vi "DAQ Loop.vi"(8 "error in":errorcluster, 10 "Queues":T1, 11 "Notifiers":T2) -> (0 "error out":errorcluster)   [LabVIEW 2014, in "DAQ.lvlib"]
uses:
  DAQ.lvlib
  support/Message Queue/Message Queue.lvlib
  TypeDefs/DAQ data.ctl
  <vilib>/ErrorRing/Error Ring.xnode
  PLC/PLC.lvlib
  support/Global names.vi
  <vilib>/Utility/error.llb/Error Cluster From Error Code.vi
  support/Message Queue/Message Cluster.ctl
  support/Notifiers/Notifiers.ctl
  Support/Notifiers/Notifiers.lvlib
  support/Message Queue/All Message Queues.ctl
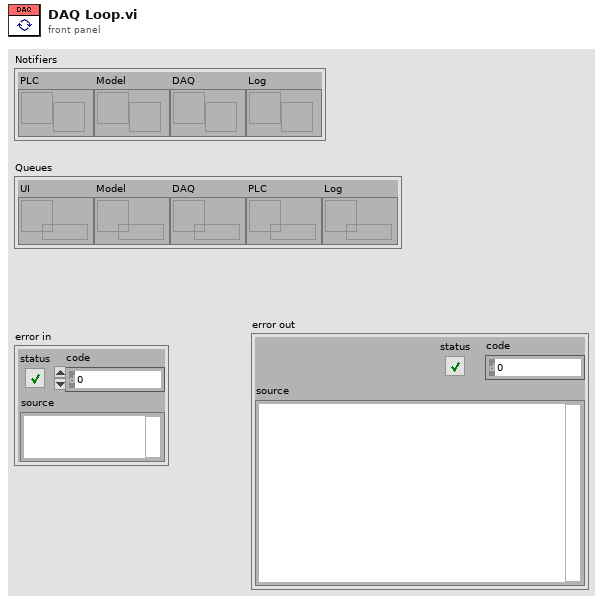
[diagram p1: front panel]
types:
  T1 = typedef "Message Queue.lvlib/All Message Queues.ctl" = cluster{"UI":refnum<queue>, "Model":refnum<queue>, "DAQ":refnum<queue>, "PLC":refnum<queue>, "Log":refnum<queue>}
  T2 = typedef "Notifiers.lvlib/Notifiers.ctl" = cluster{"PLC":refnum<notifier>, "Model":refnum<notifier>, "DAQ":refnum<notifier>, "Log":refnum<notifier>}
  T3 = typedef "DAQ.lvlib/DAQ data.ctl" = cluster{"Power switch (DI)":cluster{"Channel":tag, "Data":bool}, "Dispose barrel (DI)":cluster{"Channel":tag, "Data":bool}, "Pump status (DO)":cluster{"Channel":tag, "Data":bool}, "Barrel position (AI)":cluster{"Channel":tag, "Data":dbl}}
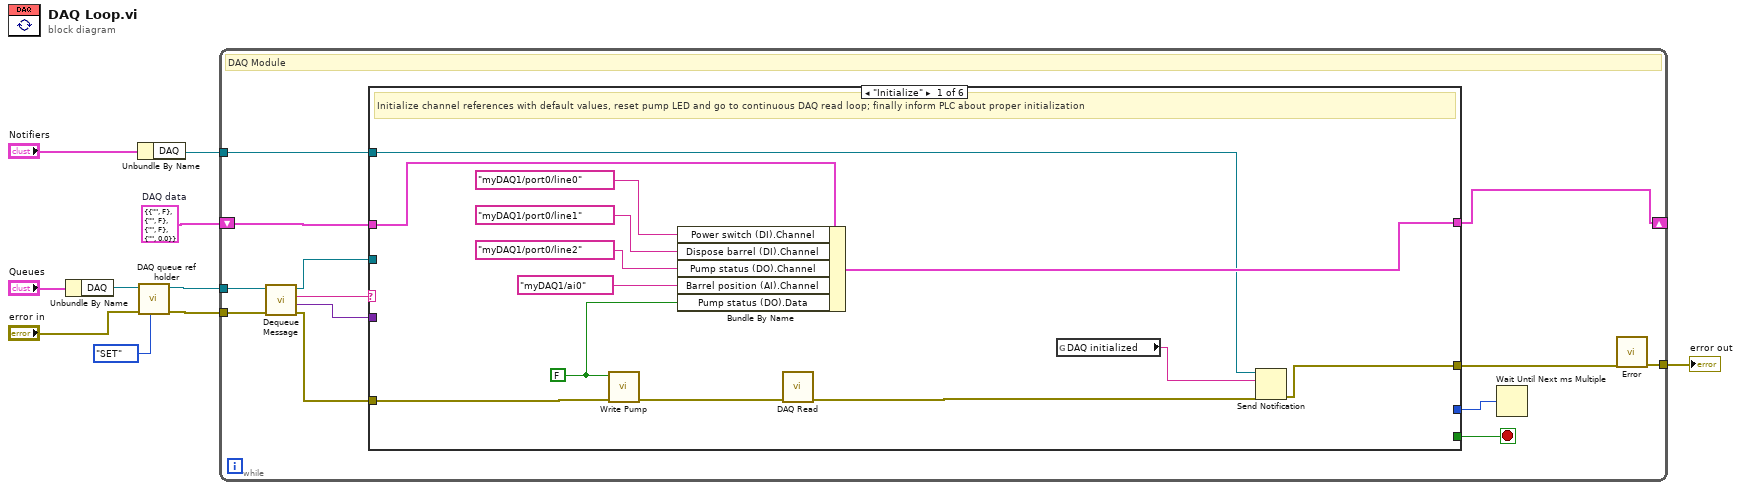
[diagram p0: block diagram]
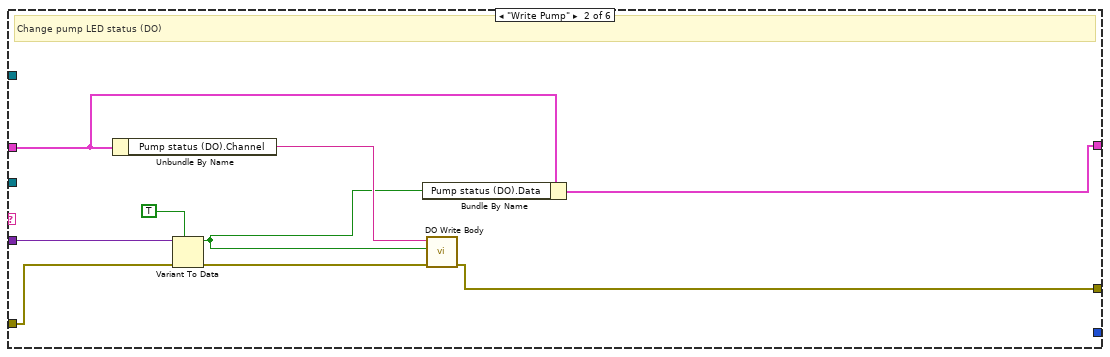
[diagram p2: hidden frame]
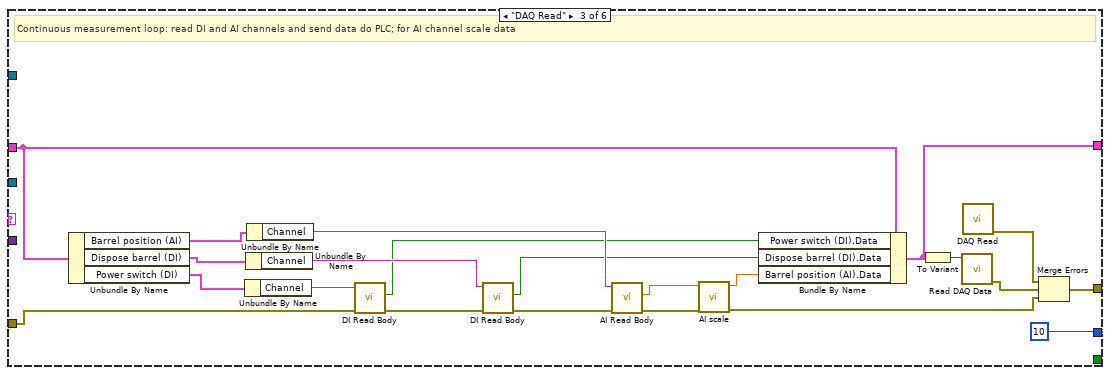
[diagram p3: hidden frame]
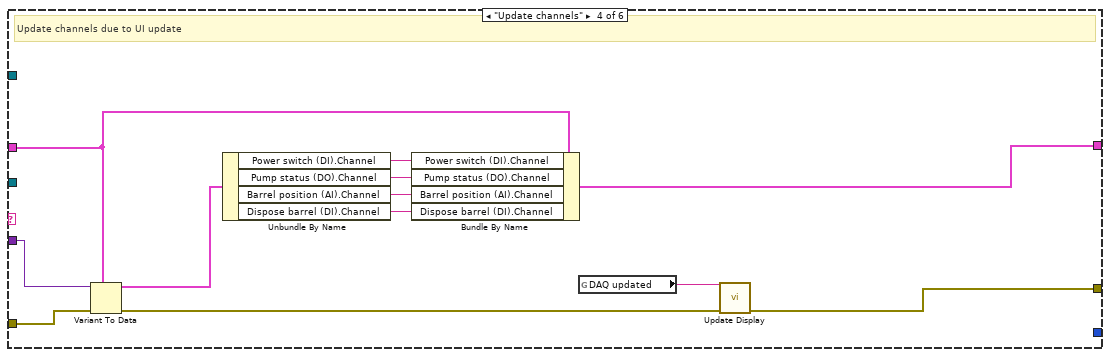
[diagram p4: hidden frame]
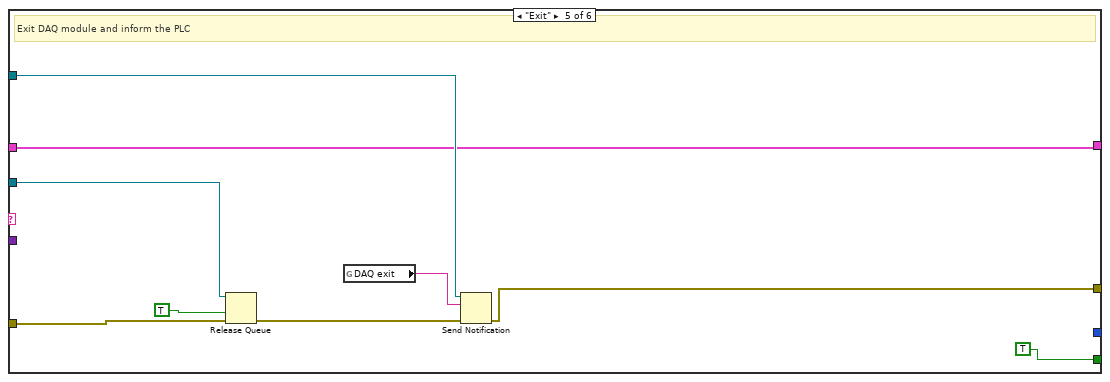
[diagram p5: hidden frame]
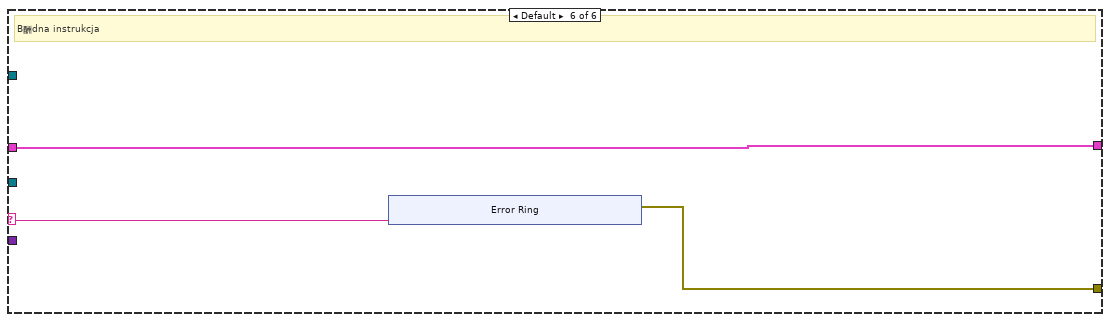
[diagram p6: hidden frame]
diagram:
  w10 = T3 {"Power switch (DI)"={"Channel"="", "Data"=FALSE}, "Dispose barrel (DI)"={"Channel"="", "Data"=FALSE}, "Pump status (DO)"={"Channel"="", "Data"=FALSE}, "Barrel position (AI)"={"Channel"="", "Data"=0.0}}  # DAQ data
  n1 = Unbundle By Name("Queues") -> ("DAQ"=w5:refnum<queue>)
  n2 = Unbundle By Name("Notifiers") -> ("DAQ"=w6:refnum<notifier>)
  n3 = call "DAQ queue ref holder.vi"("Action"=enum16{"GET", "SET"}."SET", "error in"="error in", "Message Queue In"=w5) -> ("error out"=w3:errorcluster, "Input Message Queue"=w4:refnum<queue>)  [unwired: 7 in]
  n4 = while {
    tunnel: w3 -> [w23]
    tunnel: w4 -> [w11]
    tunnel: w6 -> [w19]
    shift-right: [w18] -> _
    shift-left: w10 -> [w16]
    tunnel: [w14] -> w8
    stop <- w20 stop-if-true
    # "DAQ Module"
    n5 = call "Dequeue Message.vi"("error in (no error)"=w23, "Message Queue"=w11) -> ("error out"=w22:errorcluster, "Message Data"=w21:variant, "Message"=w12:string, "dup Message Queue"=w13:refnum<queue>)  [unwired: 6 in]
    n6 = case shown="\"Initialize\"" w12 {
      selector: w12 -> [_ _ _ _ _ w90]
      tunnel: w22 -> [w29 w45 w54 w78 w82 _]
      tunnel: [w35 w37 w49 w70 w81 w89] -> w15
      tunnel: w21 -> [_ w44 _ w79 _ _]
      tunnel: [_ _ _ _ TRUE _] -> w20
      tunnel: w13 -> [_ _ _ _ w88 _]
      tunnel: w19 -> [w27 _ _ _ w87 _]
      tunnel: w16 -> [w34 w41 w64 w77 w83 w91]
      tunnel: [w33 w43 w58 w72 w83 w91] -> w18
      tunnel: [_ _ u32 10 ("millisecond multiple") _ _ _] -> w17
      frame "Initialize" {
        w26 = FALSE
        # "Initialize channel references with default values, reset pump LED and go to continuous DAQ read loop; finally inform PLC about proper initialization"
        n7 = call "Write Pump.vi"("error in"=w29, "Pump state"=w26) -> ("error out"=w28:errorcluster)  [unwired: 9 in]
        n8 = Bundle By Name(cluster=w34, "Power switch (DI).Channel"=tag "myDAQ1/port0/line0", "Dispose barrel (DI).Channel"=tag "myDAQ1/port0/line1" ("Power switch (DI).Channel"), "Pump status (DO).Channel"=tag "myDAQ1/port0/line2" ("Power switch (DI).Channel"), "Barrel position (AI).Channel"=tag "myDAQ1/ai0", "Pump status (DO).Data"=w26) -> (w33:T3)
        n9 = call "DAQ Read.vi"("error in"=w28) -> ("error out"=w25:errorcluster)  [unwired: 10 in]
        n10 = global read "Global names.vi" "DAQ initialized"() -> (w24:string)
        n11 = Send Notification(notification=w24, notifier=w27, error in (no error)=w25) -> (error out=w35:errorcluster)  [unwired: 1 out]
      }
      frame "Write Pump" {
        # "Change pump LED status (DO)"
        n12 = Unbundle By Name(w41) -> ("Pump status (DO).Channel"=w42:tag)
        n13 = Variant To Data(error in=w45, type=TRUE, Variant=w44) -> (data=w39:bool, error out=w38:errorcluster)
        n14 = Bundle By Name(cluster=w41, "Pump status (DO).Data"=w39) -> (w43:T3)
        n15 = call "DO Write Body.vi"("error in"=w38, "data"=w39, "Channel"=w42) -> ("error out"=w37:errorcluster)  [unwired: 6 in]
      }
      frame "DAQ Read" {
        # "Continuous measurement loop: read DI and AI channels and send data do PLC; for AI channel scale data"
        n16 = Unbundle By Name(w64) -> ("Barrel position (AI)"=w51:cluster{"Channel":tag, "Data":dbl}, "Dispose barrel (DI)"=w52:cluster{"Channel":tag, "Data":bool}, "Power switch (DI)"=w53:cluster{"Channel":tag, "Data":bool})
        n17 = Unbundle By Name(w53) -> ("Channel"=w63:tag)
        n18 = Unbundle By Name(w52) -> ("Channel"=w62:tag)
        n19 = Unbundle By Name(w51) -> ("Channel"=w61:tag)
        n20 = call "DI Read Body.vi"("error in"=w54, "Channel"=w63) -> ("error out"=w67:errorcluster, "data"=w56:bool)  [unwired: 6 in]
        n21 = call "DI Read Body.vi"("error in"=w67, "Channel"=w62) -> ("error out"=w66:errorcluster, "data"=w57:bool)  [unwired: 6 in]
        n22 = call "AI Read Body.vi"("error in"=w66, "Channel"=w61) -> ("error out"=w50:errorcluster, "data"=w65:dbl)  [unwired: 6 in]
        n23 = call "AI scale.vi"("error in"=w50, "Data in"=w65) -> ("error out"=w46:errorcluster, "Data out"=w60:dbl)  [unwired: 8 in]
        n24 = Bundle By Name(cluster=w64, "Power switch (DI).Data"=w56, "Dispose barrel (DI).Data"=w57, "Barrel position (AI).Data"=w60) -> (w58:T3)
        n25 = To Variant(anything=w58) -> (Variant=w55:variant)
        n26 = call "Read DAQ Data.vi"("Message Data"=w55) -> ("error out"=w47:errorcluster)  [unwired: 10 in]
        n27 = call "DAQ Read.vi"() -> ("error out"=w48:errorcluster)  [unwired: 11 in]
        n28 = Merge Errors(w48, w47, w46) -> (w49:errorcluster)
      }
      frame "Update channels" {
        # "Update channels due to UI update"
        n29 = Variant To Data(error in=w78, type=w77, Variant=w79) -> (data=w69:T3, error out=w71:errorcluster)
        n30 = Unbundle By Name(w69) -> ("Power switch (DI).Channel"=w76:tag, "Pump status (DO).Channel"=w75:tag, "Barrel position (AI).Channel"=w74:tag, "Dispose barrel (DI).Channel"=w73:tag)
        n31 = Bundle By Name(cluster=w77, "Power switch (DI).Channel"=w76, "Pump status (DO).Channel"=w75, "Barrel position (AI).Channel"=w74, "Dispose barrel (DI).Channel"=w73) -> (w72:T3)
        n32 = global read "Global names.vi" "DAQ updated"() -> (w68:string)
        n33 = call "Update Display.vi"("error in"=w71, "Message string"=w68) -> ("error out"=w70:errorcluster)  [unwired: 9 in]
      }
      frame "Exit" {
        # "Exit DAQ module and inform the PLC"
        n34 = Release Queue(queue=w88, force destroy? (F)=TRUE, error in (no error)=w82) -> (error out=w86:errorcluster)  [unwired: 2 out]
        n35 = global read "Global names.vi" "DAQ exit"() -> (w80:string)
        n36 = Send Notification(notification=w80, notifier=w87, error in (no error)=w86) -> (error out=w81:errorcluster)  [unwired: 1 out]
      }
      frame Default {
        # "B酬dna instrukcja"
        n37 = xnode "Error Ring"("parameter 0"=w90) -> ("error out"=w89:errorcluster)
      }
    }
    n38 = Wait Until Next ms Multiple(millisecond multiple=w17) -> ()  [unwired: 1 out]
    n39 = call "Error.vi"("error in"=w15) -> ("error out"=w14:errorcluster)  [unwired: 10 in]
  }
  "error out" <- w8
